vi "AssertArrayDimension_3DArray-CSG.vi"(11 "Array in":csg[][][](array[numeric])) -> (3 "Array out":csg[][][](array[numeric]))   [LabVIEW 2020, in "OpenLvVision_OpenCv.lvlib"]
doc: "Assert array dimension.\nNo malleable to breake vi inlining!"
uses:
  OpenLvVision_OpenCv.lvlib
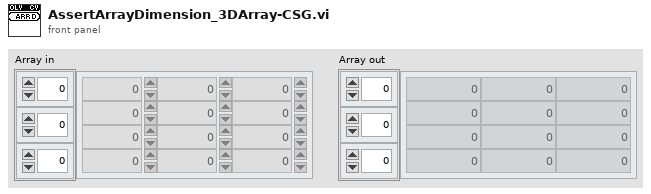
[diagram p1: front panel]
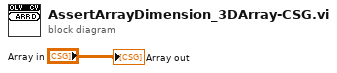
[diagram p0: block diagram]
diagram:
  "Array out" <- "Array in"
